vi "File Column Headers.vi"() -> (3 "Column Header":string[][](array[string]))   [LabVIEW 2017]
uses:
  TCP/TCP Engine/SubVIs/SubVI - Global.vi
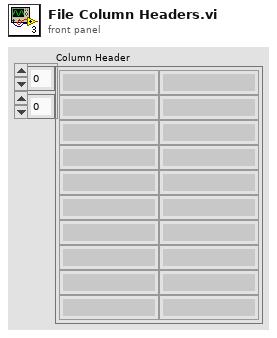
[diagram p1: front panel]
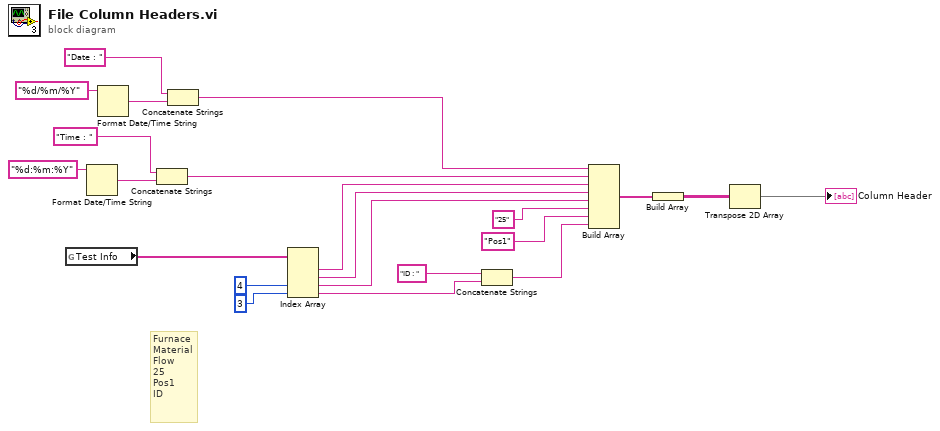
[diagram p0: block diagram]
diagram:
  # "Furnace\nMaterial\nFlow\n25\nPos1\nID"
  n1 = global read "SubVI - Global.vi" "Test Info"() -> (w15:string[])
  n2 = Format Date/Time String(time format string (%c)="%d:%m:%Y") -> (date/time string=w18:string)  [unwired: 2 in]
  n3 = Format Date/Time String(time format string (%c)="%d/%m/%Y") -> (date/time string=w19:string)  [unwired: 2 in]
  n4 = Concatenate Strings("Time : ", w18) -> (w13:string)
  n5 = Concatenate Strings("Date : ", w19) -> (w14:string)
  n6 = Index Array(array=w15, index #3=4 ("index"), index #4=3 ("index")) -> (element #1=w12:string, element #2=w11:string, element #3=w7:string, element #4=w4:string)  [unwired: 2 in]
  n7 = Concatenate Strings("ID : " ("element"), w4) -> (w3:string)
  n8 = Build Array(w14, w13, w12, w11, w7, "25" ("element"), "Pos1" ("element"), w3) -> (w22:string[])
  n9 = Build Array(w22) -> (w2:string[][])
  n10 = Transpose 2D Array(2D array=w2) -> (transposed array=→"Column Header":string[][])
